vi "Read Server Configuration.vi"(8 "error in (no error)":errorcluster, 10 "server index":u16, 11 "PLBB in":refnum<class "PL BlackBox Modbus Client.lvclass">) -> (0 "error out":errorcluster, 2 "server configuration":T1 {"Modbus server"."protocol" items=["RTU", "ASCII", "TCP"]}, 3 "PLBB out":refnum<class "PL BlackBox Modbus Client.lvclass">)   [LabVIEW 2015, in "PL BlackBox Modbus Client.lvclass"]
doc: "Reads the server configuration."
uses:
  PL BlackBox Modbus Client.lvclass
  <vilib>/plasmapper/PL Modbus Client/PL Modbus Client.lvclass
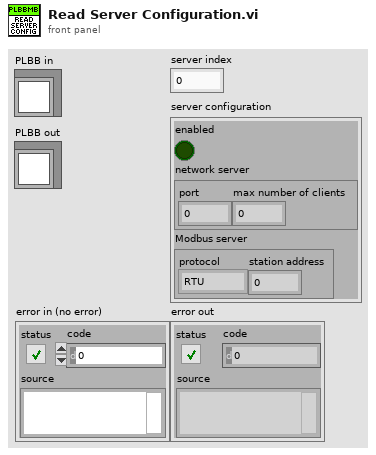
[diagram p1: front panel]
types:
  T1 = cluster{"enabled":bool, "network server":cluster{"port":u16, "max number of clients":u16}, "Modbus server":cluster{"protocol":u16, "station address":u16}}
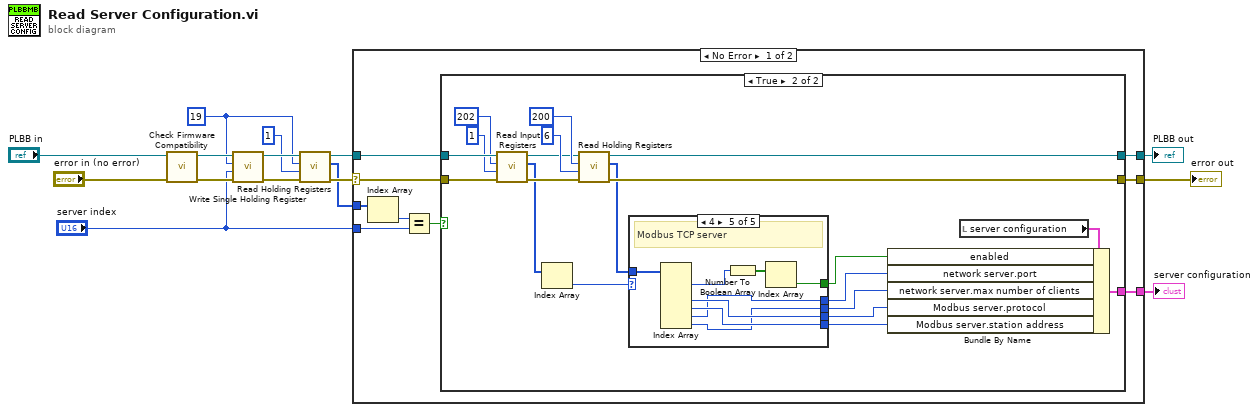
[diagram p0: block diagram]
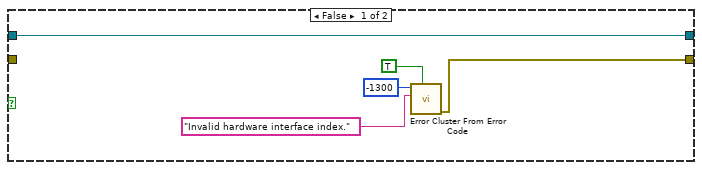
[diagram p2: hidden frame]
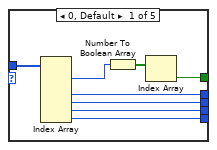
[diagram p3: hidden frame]
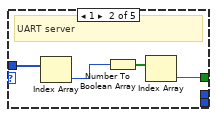
[diagram p4: hidden frame]
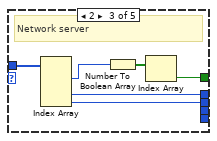
[diagram p5: hidden frame]
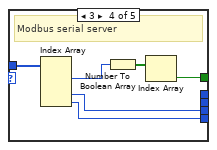
[diagram p6: hidden frame]
diagram:
  w7 = u16 19 ("address")
  n1 = call-dynamic "Check Firmware Compatibility.vi"("error in (no error)"="error in (no error)", "PLBB in"="PLBB in") -> ("error out"=w10:errorcluster, "PLBB out"=w11:refnum<class "PL BlackBox Modbus Client.lvclass">)  [unwired: 8 in]
  n2 = call <vilib>:"Write Single Holding Register.vi"("error in (no error)"=w10, "value"="server index", "address"=w7, "MODBUS in"=w11) -> ("error out"=w6:errorcluster, "MODBUS out"=w9:refnum<class "PL BlackBox Modbus Client.lvclass">)  [unwired: 6 in]
  n3 = call <vilib>:"Read Holding Registers.vi"("error in (no error)"=w6, "number of holding registers"=u16 1 ("address"), "address"=w7, "MODBUS in"=w9) -> ("error out"=w5:errorcluster, "values"=w3:u16[], "MODBUS out"=w4:refnum<class "PL BlackBox Modbus Client.lvclass">)  [unwired: 5 in]
  n4 = case shown="No Error" w5 {
    selector: w5 -> [w17 w82]
    tunnel: [w24 w82] -> w15
    tunnel: [w23 w83] -> w14
    tunnel: w4 -> [w18 w83]
    tunnel: w3 -> [w22 _]
    tunnel: "server index" -> [w20 _]
    tunnel: [w16 _] -> w1
    frame No Error {
      n5 = Index Array(array=w22) -> (element=w21:u16)  [unwired: 1 in]
      n6 = Equal?(x=w21, y=w20) -> (x = y?=w19:bool)
      n7 = case shown="True" w19 {
        tunnel: [w25 w49] -> w24
        tunnel: [w29 w48] -> w23
        tunnel: w18 -> [w29 w40]
        tunnel: w17 -> [_ w39]
        tunnel: [_ w44] -> w16
        frame False {
          n8 = call <vilib>:"Error Cluster From Error Code.vi"("show call chain? (False)"=TRUE, "error message (\"\")"="Invalid hardware interface index." ("error message (\"\")"), "error code (0)"=-1300) -> ("error out"=w25:errorcluster)  [unwired: 6 in]
        }
        frame True {
          n9 = call <vilib>:"Read Input Registers.vi"("error in (no error)"=w39, "number of input registers"=u16 1 ("address"), "address"=u16 202, "MODBUS in"=w40) -> ("error out"=w38:errorcluster, "values"=w34:u16[], "MODBUS out"=w37:refnum<class "PL BlackBox Modbus Client.lvclass">)  [unwired: 5 in]
          n10 = Index Array(array=w34) -> (element=w31:u16)  [unwired: 1 in]
          n11 = call <vilib>:"Read Holding Registers.vi"("error in (no error)"=w38, "number of holding registers"=u16 6 ("address"), "address"=u16 200, "MODBUS in"=w37) -> ("error out"=w49:errorcluster, "values"=w43:u16[], "MODBUS out"=w48:refnum<class "PL BlackBox Modbus Client.lvclass">)  [unwired: 5 in]
          n12 = case shown="4" w31 {
            tunnel: w43 -> [w57 w61 w67 w73 w81]
            tunnel: [w56 _ w66 _ w78] -> w42
            tunnel: [w55 _ w65 _ w77] -> w41
            tunnel: [w54 _ _ w71 w79] -> w33
            tunnel: [w53 _ _ w72 w80] -> w32
            tunnel: [w51 w58 w63 w69 w75] -> w30
            frame 0, Default {
              n13 = Index Array(array=w57) -> (element #1=w50:u16, element #3=w56:u16, element #4=w55:u16, element #5=w54:u16, element #6=w53:u16)  [unwired: 6 in, 1 out]
              n14 = Number To Boolean Array(number=w50) -> (Boolean array=w52:bool[])
              n15 = Index Array(array=w52) -> (element=w51:bool)  [unwired: 1 in]
            }
            frame 1 {
              # "UART server"
              n16 = Index Array(array=w61) -> (element=w59:u16)  [unwired: 1 in]
              n17 = Number To Boolean Array(number=w59) -> (Boolean array=w60:bool[])
              n18 = Index Array(array=w60) -> (element=w58:bool)  [unwired: 1 in]
            }
            frame 2 {
              # "Network server"
              n19 = Index Array(array=w67) -> (element #1=w62:u16, element #3=w66:u16, element #4=w65:u16)  [unwired: 4 in, 1 out]
              n20 = Number To Boolean Array(number=w62) -> (Boolean array=w64:bool[])
              n21 = Index Array(array=w64) -> (element=w63:bool)  [unwired: 1 in]
            }
            frame 3 {
              # "Modbus serial server"
              n22 = Index Array(array=w73) -> (element #1=w68:u16, element #3=w71:u16, element #4=w72:u16)  [unwired: 4 in, 1 out]
              n23 = Number To Boolean Array(number=w68) -> (Boolean array=w70:bool[])
              n24 = Index Array(array=w70) -> (element=w69:bool)  [unwired: 1 in]
            }
            frame 4 {
              # "Modbus TCP server"
              n25 = Index Array(array=w81) -> (element #1=w74:u16, element #3=w79:u16, element #4=w80:u16, element #5=w78:u16, element #6=w77:u16)  [unwired: 6 in, 1 out]
              n26 = Number To Boolean Array(number=w74) -> (Boolean array=w76:bool[])
              n27 = Index Array(array=w76) -> (element=w75:bool)  [unwired: 1 in]
            }
          }
          n28 = local read "server configuration"() -> (w45:T1)
          n29 = Bundle By Name(cluster=w45, "enabled"=w30, "network server.port"=w42, "network server.max number of clients"=w41, "Modbus server.protocol"=w33, "Modbus server.station address"=w32) -> (w44:T1)
        }
      }
    }
    frame Error {
    }
  }
  "error out" <- w15
  "PLBB out" <- w14
  "server configuration" <- w1
